vi "Verification.vi"(5 "verification":bool=TRUE, 7 "Motor\n(man/auto)":bool, 8 "error in (no error)":errorcluster, 10 "Value in":variant, 11 "AISAS motor in":refnum<class "AISAS motor.lvclass">) -> (0 "error out":errorcluster, 2 "Motor":T2, 3 "AISAS motor out":refnum<class "AISAS motor.lvclass">)   [LabVIEW 2014, in "AISAS motor.lvclass"]
uses:
  motor/AISAS motor.lvclass
  Controls/Diffuser.ctl
  Controls/focus.ctl
  Controls/motor.ctl
  Controls/Rotation.ctl
  motor/AISAS motor.lvclass/AISAS motor.ctl
panel:
  in  "Rotation":T1 caption="New Value" min=0.0 max=360.0 step=1.0 format="%.1f"
  in  "Focus":T3=70.0 caption="New Value" min=70.0 max=152.0 format="%.2f"
  out "Old value":string
  out "String":string
  in  "Diffuser":T4=enum."In Beam" caption="New Value"
  in  "OK":bool
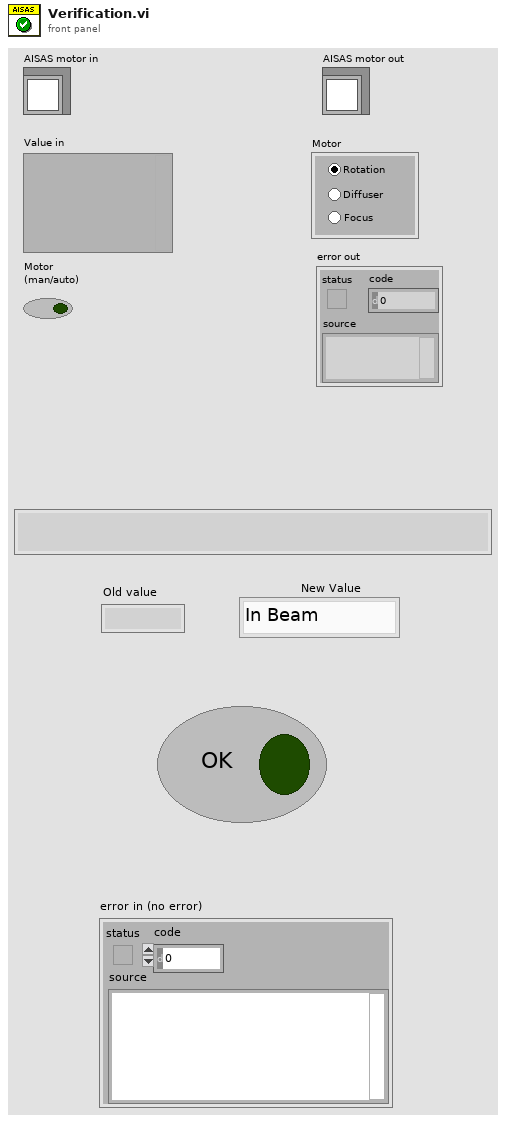
[diagram p1: front panel]
types:
  T1 = typedef "Rotation.ctl" = dbl
  T2 = typedef "motor.ctl" = enum32{"Rotation", "Diffuser ", "Focus"}
  T3 = typedef "focus.ctl" = dbl
  T4 = typedef "Diffuser.ctl" = enum16{"Out of Beam", "In Beam"}
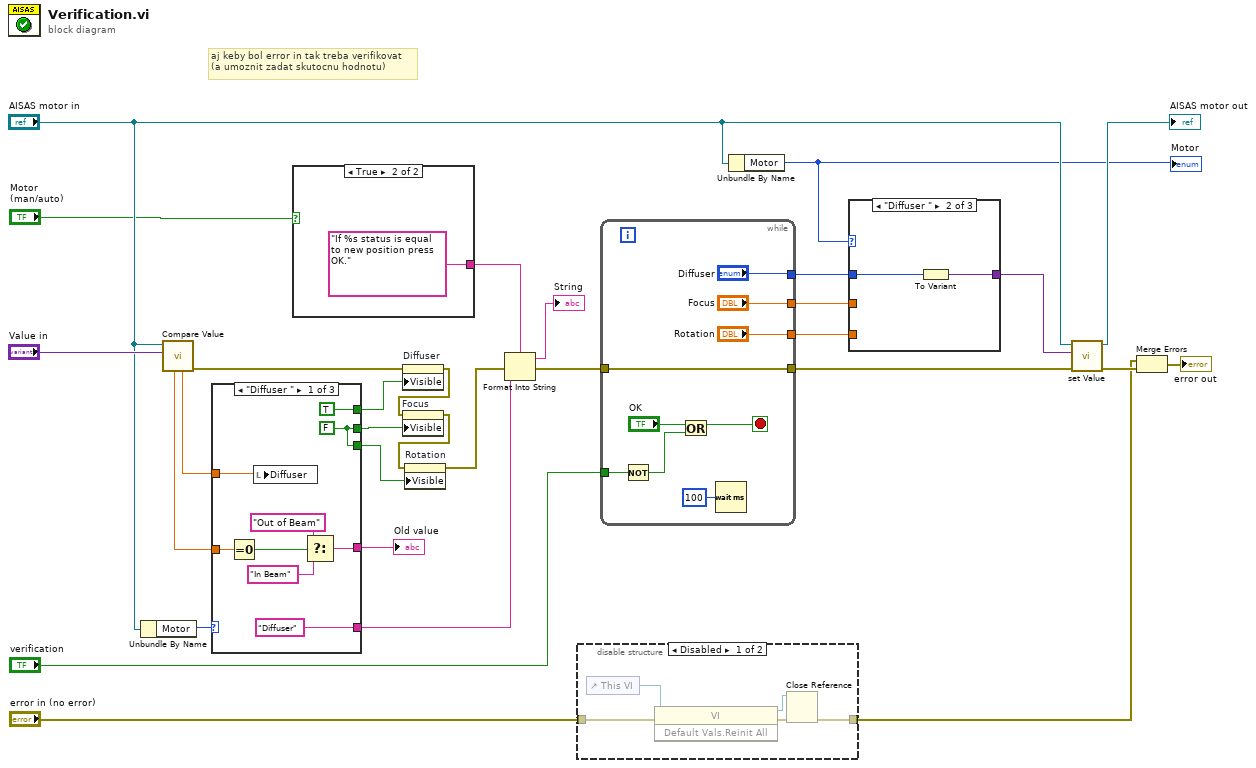
[diagram p0: block diagram]
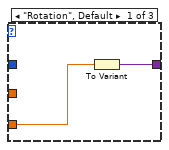
[diagram p3: hidden frame]
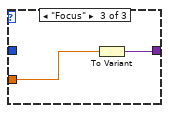
[diagram p4: hidden frame]
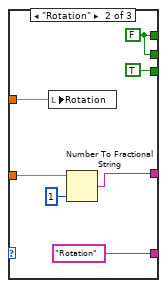
[diagram p5: hidden frame]
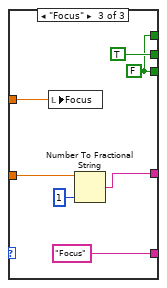
[diagram p6: hidden frame]
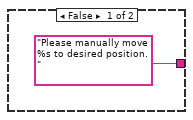
[diagram p7: hidden frame]
diagram:
  # "aj keby bol error in tak treba verifikovat\n(a umoznit zadat skutocnu hodnotu)"
  n1 = Unbundle By Name("AISAS motor in") -> ("Motor"=w25:T2)
  n2 = call "Compare Value.vi"("new Value"="Value in", "AISAS motor in"="AISAS motor in") -> ("error out"=w18:errorcluster, "new value"=w21:dbl, "old value"=w20:dbl)  [unwired: 4 in, 3 out]
  n3 = case shown="\"Diffuser \"" w25 {
    tunnel: ["Diffuser" "Rotation" "Focus"] -> w17
    tunnel: w21 -> [w38 w40 w52]
    tunnel: w20 -> [w37 w44 w48]
    tunnel: [w33 w43 w47] -> w19
    tunnel: [w31 w41 TRUE ("Visible")] -> w11
    tunnel: [TRUE ("Visible") w41 w50] -> w10
    tunnel: [w31 TRUE ("Visible") w50] -> w6
    frame "Diffuser " {
      w31 = FALSE ("Visible")
      n4 = Equal To 0?(x=w37) -> (x = 0?=w36:bool)
      n5 = local write "Diffuser"(w38) -> ()
      n6 = Select(t="Out of Beam", s=w36, f="In Beam") -> (s? t:f=w33:string)
    }
    frame "Rotation" {
      w41 = FALSE ("Visible")
      n7 = local write "Rotation"(w40) -> ()
      n8 = Number To Fractional String(number=w44, precision (6)=i16 1) -> (F-format string=w43:string)  [unwired: 2 in]
    }
    frame "Focus" {
      w50 = FALSE ("Visible")
      n9 = local write "Focus"(w52) -> ()
      n10 = Number To Fractional String(number=w48, precision (6)=i16 1) -> (F-format string=w47:string)  [unwired: 2 in]
    }
  }
  "Old value" <- w19
  n11 = case shown="True" "Motor\n(man/auto)" {
    tunnel: ["Please manually move %s to desired position." ("String") "If %s status is equal to new position press OK." ("String")] -> w23
    frame False {
    }
    frame True {
    }
  }
  n12 = property on="Diffuser" class="Enum (strict)"(error in=w18, "Visible"=w10) -> (error out=w12:errorcluster)  [unwired: 1 in, 1 out]
  n13 = property on="Focus" class="DigNum (strict)"(error in=w12, "Visible"=w11) -> (error out=w5:errorcluster)  [unwired: 1 in, 1 out]
  n14 = property on="Rotation" class="DigNum (strict)"(error in=w5, "Visible"=w6) -> (error out=w7:errorcluster)  [unwired: 1 in, 1 out]
  n15 = Format Into String(format string=w23, error in=w7, w17) -> (resulting string=→"String":string, error out=w24:errorcluster)  [unwired: 1 in]
  n16 = disable-structure shown="Disabled" {
    disable-tunnel: "error in (no error)" -> [w57 w61]
    disable-tunnel: [w56 w61] -> w2
    frame Disabled {
      n17 = control-ref of="This VI"() -> (w60:refnum<vi>)
      n18 = invoke class="VI" method="Default Vals.Reinit All"(reference=w60, error in=w57) -> (reference out=w58:refnum<vi>, error out=w59:errorcluster)  [unwired: 1 in, 1 out]
      n19 = Close Reference(reference=w58, error in (no error)=w59) -> (error out=w56:errorcluster)
    }
    frame Enabled {
    }
  }
  n20 = while {
    tunnel: w24 -> [w69]
    tunnel: [w69] -> w13
    tunnel: ["Diffuser"] -> w16
    tunnel: ["Focus"] -> w15
    tunnel: ["Rotation"] -> w14
    tunnel: "verification" -> [w63]
    stop <- w64 stop-if-true
    n21 = Not(x=w63) -> (.not. x?=w62:bool)
    n22 = Or(x="OK", y=w62) -> (x .or. y?=w64:bool)
    n23 = Wait (ms)(milliseconds to wait=u32 100) -> ()  [unwired: 1 out]
  }
  n24 = Unbundle By Name("AISAS motor in") -> ("Motor"=w27:T2)
  "Motor" <- w27
  n25 = case shown="\"Diffuser \"" w27 {
    tunnel: w16 -> [_ w74 _]
    tunnel: w15 -> [_ _ w76]
    tunnel: w14 -> [w71 _ _]
    tunnel: [w72 w73 w75] -> w4
    frame "Rotation", Default {
      n26 = To Variant(anything=w71) -> (Variant=w72:variant)
    }
    frame "Diffuser " {
      n27 = To Variant(anything=w74) -> (Variant=w73:variant)
    }
    frame "Focus" {
      n28 = To Variant(anything=w76) -> (Variant=w75:variant)
    }
  }
  n29 = call "set Value.vi"("error in (no error)"=w13, "Value"=w4, "AISAS motor in"="AISAS motor in") -> ("error out"=w9:errorcluster, "AISAS motor out"=→"AISAS motor out":refnum<class "AISAS motor.lvclass">)  [unwired: 7 in]
  n30 = Merge Errors(w2, w9) -> (→"error out":errorcluster)
